vi "Wait for Acquisition Complete.vi"(8 "error in (no error)":errorcluster, 9 "Maximum Time (10000 ms)":u32=10000, 11 "VISA resource name":refnum<visa-resource-name>) -> (0 "error out":errorcluster, 3 "VISA resource name out":refnum<visa-resource-name>)   [LabVIEW 2021, in "Agilent N6900 N7900 Series.lvlib"]
doc: "Waits for the current waveform acquisition to finish. \n\nNote:\nUse this VI only with other low-level VIs. The high-level VIs automatically incorporate this functionality. This VI does not check the instrument status."
uses:
  <instrlib>/Agilent N6900 N7900 Series/Agilent N6900 N7900 Series.lvlib
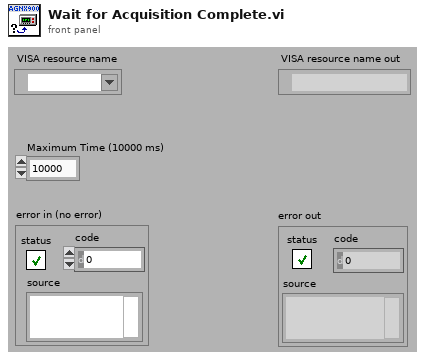
[diagram p1: front panel]
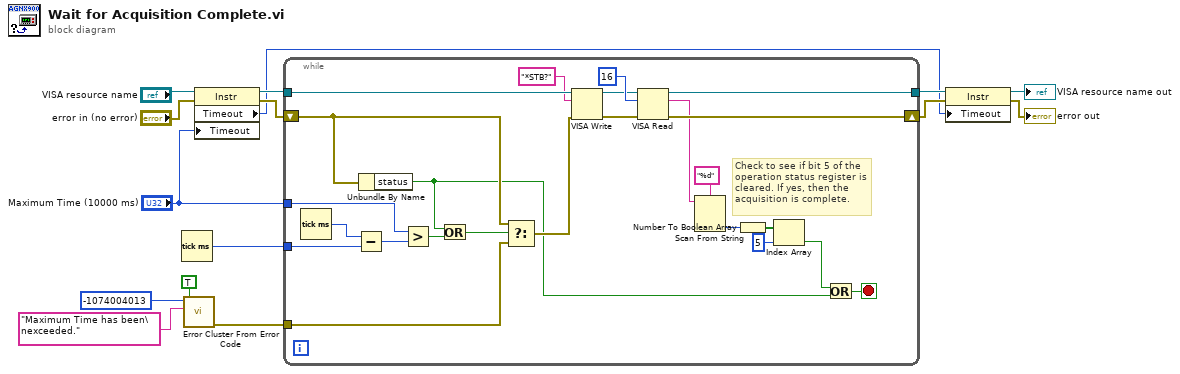
[diagram p0: block diagram]
diagram:
  n1 = Tick Count (ms)() -> (millisecond timer value=w15:u32)
  n2 = call <vilib>:"Error Cluster From Error Code.vi"("show call chain? (False)"=TRUE, "error message (\"\")"="Maximum Time has been\nexceeded." ("error message (\"\")"), "error code (0)"=-1074004013) -> ("error out"=w11:errorcluster)  [unwired: 6 in]
  n3 = property class="Instr"(reference="VISA resource name", error in="error in (no error)", "Timeout"="Maximum Time (10000 ms)") -> (reference out=w4:refnum<visa-resource-name>, error out=w3:errorcluster, "Timeout"=w2:u32)
  n4 = while {
    tunnel: [w38] -> w7
    tunnel: w4 -> [w37]
    tunnel: "Maximum Time (10000 ms)" -> [w33]
    tunnel: w15 -> [w34]
    tunnel: w11 -> [w29]
    shift-right: [w39] -> w5
    shift-left: w3 -> [w30]
    stop <- w26 stop-if-true
    # "Check to see if bit 5 of the operation status register is cleared. If yes, then the acquisition is complete."
    n5 = Tick Count (ms)() -> (millisecond timer value=w36:u32)
    n6 = Subtract(x=w36, y=w34) -> (x-y=w35:u32)
    n7 = Unbundle By Name(w30) -> ("status"=w25:bool)
    n8 = Greater?(x=w33, y=w35) -> (0:w32:bool)
    n9 = Or(x=w25, y=w32) -> (x .or. y?=w31:bool)
    n10 = Select(t=w30, s=w31, f=w29) -> (s? t:f=w28:errorcluster)
    n11 = VISA Write(VISA resource name=w37, write buffer="*STB?", error in (no error)=w28) -> (VISA resource name out=w19:refnum<visa-resource-name>, error out=w20:errorcluster)  [unwired: 1 out]
    n12 = VISA Read(VISA resource name=w19, byte count=u32 16, error in (no error)=w20) -> (VISA resource name out=w38:refnum<visa-resource-name>, read buffer=w24:string, error out=w39:errorcluster)  [unwired: 1 out]
    n13 = Scan From String(format string="%d", input string=w24) -> (output 1=w16:i32)  [unwired: 3 in, 3 out]
    n14 = Number To Boolean Array(number=w16) -> (Boolean array=w18:bool[])
    n15 = Index Array(array=w18, index=5) -> (element=w27:bool)
    n16 = Or(x=w27, y=w25) -> (x .or. y?=w26:bool)
  }
  n17 = property class="Instr"(reference=w7, error in=w5, "Timeout"=w2) -> (reference out=→"VISA resource name out":refnum<visa-resource-name>, error out=→"error out":errorcluster)
